vi "Set Group Scalar Channel Data.vi"(6 "error in (no error)":errorcluster, 7 "scalar channel in":T2 {"Data Type" format="%.0x"}, 9 "item ref in":T1 format="%.0x") -> (0 "error out":errorcluster, 3 "built channels out":T4[](array[typedef]) {"Item Ref" format="%.0x"})   [LabVIEW 2018, in "FPGA Addon System Explorer.lvlib"]
uses:
  FPGA Addon System Explorer.lvlib
  Types/Output Scalar.ctl
  Addon Shared/Types/Data Type.ctl
  <vilib>/NI Veristand/Custom Device API/Custom Device Item Ref.ctl
  Addon Shared/Types/Register Information.ctl
  Addon Shared/FPGA Addon Shared.lvlib
  <vilib>/NI Veristand/Custom Device API/Custom Device API.lvlib
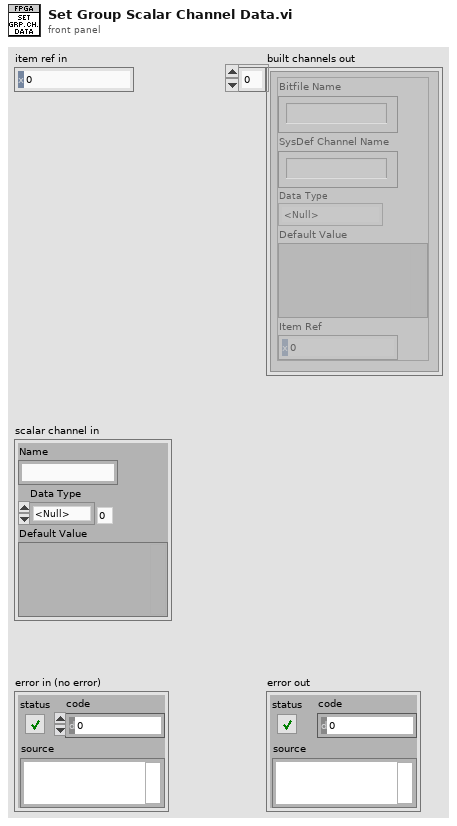
[diagram p1: front panel]
types:
  T1 = typedef "Custom Device API.lvlib/Custom Device Item Ref.ctl" = u64
  T2 = typedef "FPGA Addon Shared.lvlib/Register Information.ctl" = cluster{"Name":string, "Data Type":T3, "Default Value":variant}
  T3 = typedef "FPGA Addon Shared.lvlib/Data Type.ctl" = enum8{"<Null>", "I8", "I16", "I32", "I64", "U8", "U16", "U32", "U64", "SGL", "Boolean", "Analog PWM In Settings", "Analog PWM In", "Digital PWM In Settings", "Digital PWM In", "Digital PWM Out", "Sine Out", "FXP+/-24.5", "FXP+/-16.5", "FXP+/-32.8", "FXP+/-64.32", "FXP+/-16.7", "FXP+/-20.5", "FXP+/-27.5", "FXP+/-32.16", "FXP+16.3", "FXP+18.3", "Digital Static In", "Digital Static Out", "Digital Static In Settings", "Digital WSS Out", "Quad Encoder Settings", "Quad Encoder In", "Group"}
  T4 = typedef "FPGA Addon System Explorer.lvlib/Output Scalar.ctl" = cluster{"Bitfile Name":string, "SysDef Channel Name":string, "Data Type":T3, "Default Value":variant, "Item Ref":T1}
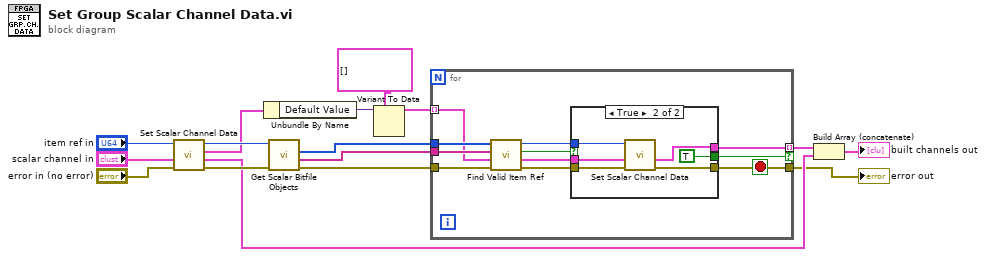
[diagram p0: block diagram]
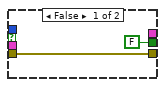
[diagram p2: hidden frame]
diagram:
  n1 = call "Set Scalar Channel Data.vi"("error in (no error)"="error in (no error)", "scalar channel in"="scalar channel in", "item ref in"="item ref in") -> ("error out"=w14:errorcluster, "built scalar channel out"=w13:T4, "scalar channel out"=w5:T2, "item ref out"=w7:T1)  [unwired: 5 in]
  n2 = Unbundle By Name(w5) -> ("Default Value"=w6:variant)
  n3 = call "Get Scalar Bitfile Objects.vi"("error in"=w14, "item ref in"=w7) -> ("error out"=w15:errorcluster, "bitfile object names"=w10:string[], "section children refs"=w8:T1[])  [unwired: 6 in, 1 out]
  n4 = Variant To Data(type=T2[] [], Variant=w6) -> (data=w9:T2[])  [unwired: 1 in, 1 out]
  n5 = for {
    tunnel: w8 -> [w24]
    tunnel: w9 -> [w22] mode=indexing
    tunnel: w10 -> [w23]
    tunnel: w15 -> [w21]
    tunnel: [w25] -> w11
    tunnel: [w27] -> w12 mode=indexing if=w26
    stop <- w25 stop-if-true
    n6 = call "Find Valid Item Ref.vi"("error in (no error)"=w21, "scalar channels"=w22, "bitfile object names"=w23, "section children refs"=w24) -> ("error out"=w20:errorcluster, "scalar channel out"=w17:T2, "found"=w19:bool, "item ref out"=w18:T1)  [unwired: 4 in]
    n7 = case shown="True" w19 {
      tunnel: w20 -> [w28 w35]
      tunnel: [w28 w34] -> w25
      tunnel: [_ w33] -> w27
      tunnel: [FALSE TRUE] -> w26
      tunnel: w18 -> [_ w31]
      tunnel: w17 -> [_ w30]
      frame False {
      }
      frame True {
        n8 = call "Set Scalar Channel Data.vi"("error in (no error)"=w35, "scalar channel in"=w30, "item ref in"=w31) -> ("error out"=w34:errorcluster, "built scalar channel out"=w33:T4)  [unwired: 5 in, 2 out]
      }
    }
  }
  "error out" <- w11
  n9 = Build Array (concatenate)(w12, w13) -> (→"built channels out":T4[])
